vi "refMgr_Example1.vi"() -> ()   [LabVIEW 2014]
uses:
  <userlib>/_NEVSTOP/TagDB/Core/TagDB.lvlib
  Util_RefMgr/RefManager(dev).lvlib
panel:
  out "::DB items::":string[](array[string])
  in  "Tab Control":enum32{"Page 1", "Page 2", "Page 3"}(tab)
  out "Waveform Chart 2":dbl(graph)
  out "Waveform Chart 3":dbl(graph)
  out "Waveform Chart 1":dbl(graph)
  in  "Combo Box":string(combo)
  out "error out":errorcluster
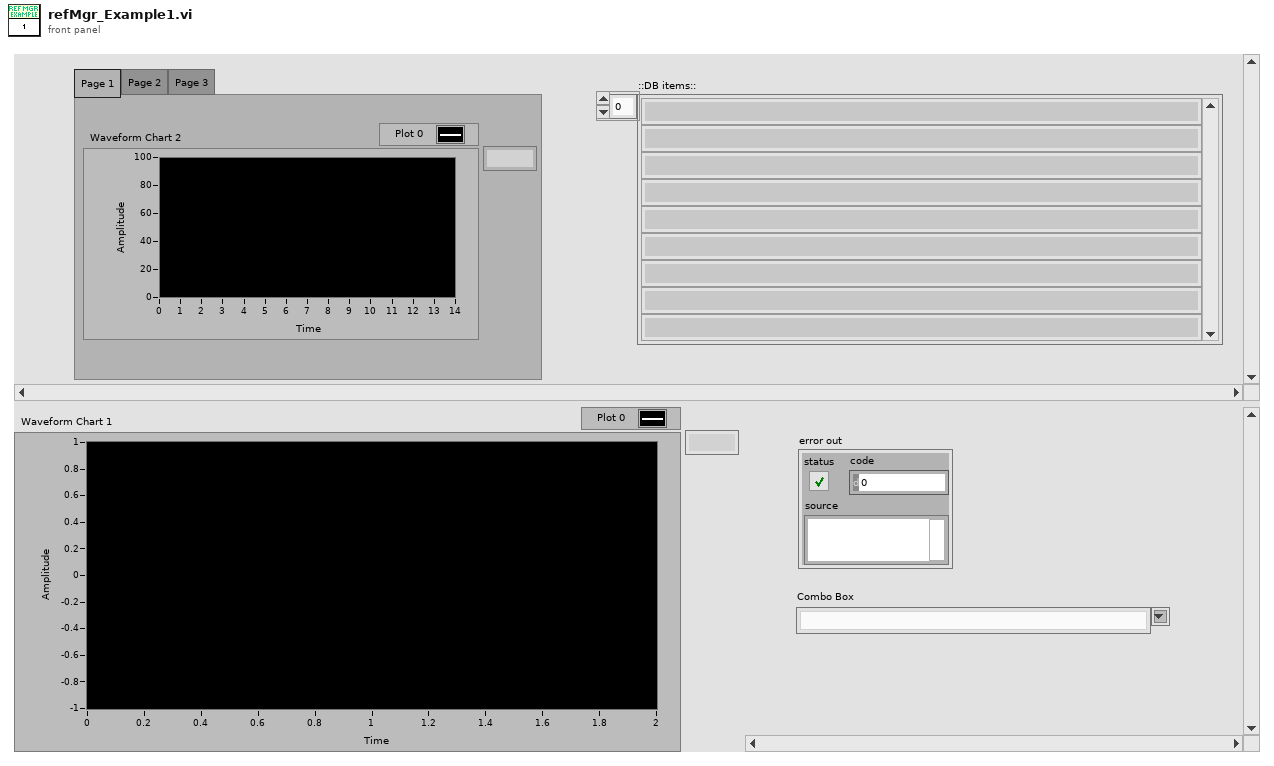
[diagram p1: front panel]
types:
  T1 = typedef "TagDB.lvlib/tagDB_Def.ctl" = refnum<k1>
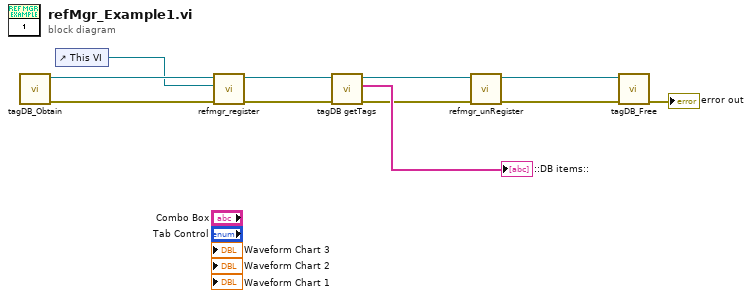
[diagram p0: block diagram]
diagram:
  n1 = call <userlib>:"tagDB_Obtain.vi"() -> ("error out"=w8:errorcluster, "DB"=w10:T1)  [unwired: 5 in, 1 out]
  n2 = control-ref of="This VI"() -> (w1:refnum<vi>)
  n3 = call "refmgr_register.vi"("error in (no error)"=w8, "VI Refnum"=w1, "TagDB in"=w10) -> ("error out"=w6:errorcluster, "TagDB out"=w9:T1)  [unwired: 6 in, 1 out]
  n4 = call <userlib>:"tagDB getTags.vi"("error in (no error)"=w6, "DB Ref in"=w9) -> ("error out"=w3:errorcluster, "DB items"=→"::DB items::":string[], "DB Ref out"=w7:T1)  [unwired: 7 in]
  n5 = call "refmgr_unRegister.vi"("error in (no error)"=w3, "TagDB in"=w7) -> ("error out"=w2:errorcluster, "TagDB out"=w4:T1)  [unwired: 8 in]
  n6 = call <userlib>:"tagDB_Free.vi"("error in (no error)"=w2, "DB Ref"=w4) -> ("error out"=→"error out":errorcluster)  [unwired: 9 in]
